vi "terminate.vi"(8 "error in (no error)":errorcluster, 11 "DL090216Display in":refnum<class "DisplayDL090216.lvclass">) -> (0 "error out":errorcluster, 3 "DL090216Display out":refnum<class "DisplayDL090216.lvclass">)   [LabVIEW 2010, in "DisplayDL090216.lvclass"]
uses:
  DisplayDL090216.lvclass
  common/classes/Image/Image/Image.lvclass
  DisplayDL090216.lvclass/DisplayDL090216.ctl
  GenericDisplay/GenericDisplay/GenericDisplay.lvclass
  common/classes/ErrorController/ErrorController/class_data.vi
  common/classes/ErrorController/ErrorController/ErrorController.lvclass
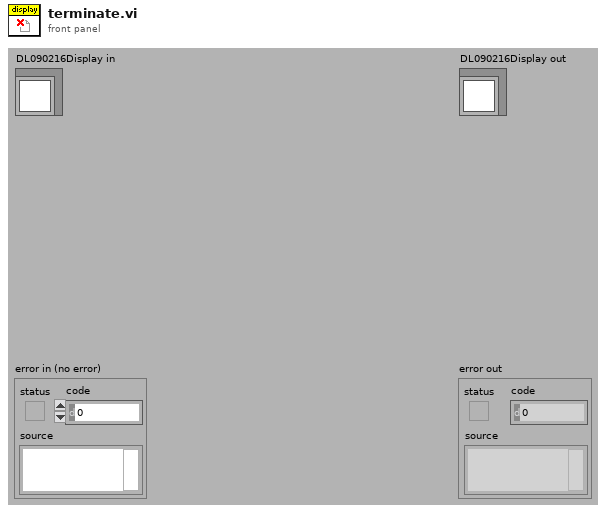
[diagram p1: front panel]
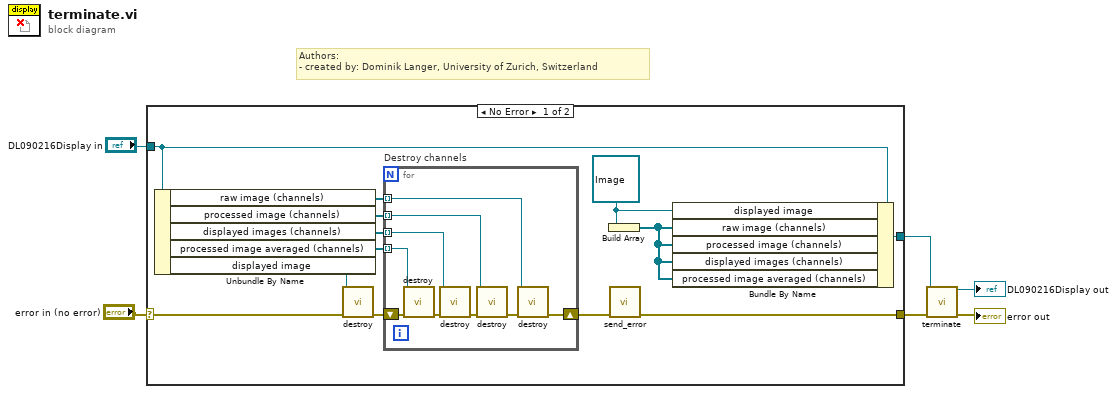
[diagram p0: block diagram]
diagram:
  # "Authors: \n- created by: Dominik Langer, University of Zurich, Switzerland"
  n1 = case shown="No Error" "error in (no error)" {
    selector: "error in (no error)" -> [w10 w30]
    tunnel: [w12 w30] -> w4
    tunnel: [w14 w29] -> w2
    tunnel: "DL090216Display in" -> [w11 w29]
    frame No Error {
      w13 = refnum<class "Image.lvclass"> refnum ("Image.lvclass")
      n2 = Unbundle By Name(w11) -> ("raw image (channels)"=w17:refnum<class "Image.lvclass">[], "processed image (channels)"=w16:refnum<class "Image.lvclass">[], "displayed images (channels)"=w15:refnum<class "Image.lvclass">[], "processed image averaged (channels)"=w8:refnum<class "Image.lvclass">[], "displayed image"=w19:refnum<class "Image.lvclass">)
      n3 = call-dynamic "destroy.vi"("error in (no error)"=w10, "Image in"=w19) -> ("error out"=w18:errorcluster)  [unwired: 9 out]
      n4 = for "Destroy channels" {
        shift-right: [w24] -> w9
        shift-left: w18 -> [w28]
        tunnel: w17 -> [w20] mode=indexing
        tunnel: w16 -> [w21] mode=indexing
        tunnel: w15 -> [w22] mode=indexing
        tunnel: w8 -> [w23] mode=indexing
        n5 = call-dynamic "destroy.vi"("error in (no error)"=w28, "Image in"=w23) -> ("error out"=w27:errorcluster)  [unwired: 9 out]
        n6 = call-dynamic "destroy.vi"("error in (no error)"=w27, "Image in"=w22) -> ("error out"=w26:errorcluster)  [unwired: 9 out]
        n7 = call-dynamic "destroy.vi"("error in (no error)"=w26, "Image in"=w21) -> ("error out"=w25:errorcluster)  [unwired: 9 out]
        n8 = call-dynamic "destroy.vi"("error in (no error)"=w25, "Image in"=w20) -> ("error out"=w24:errorcluster)  [unwired: 9 out]
      }
      n9 = Build Array(w13) -> (w7:refnum<class "Image.lvclass">[])
      n10 = call "send_error.vi"("error in (no error)"=w9) -> ("error out"=w12:errorcluster)  [unwired: 10 in]
      n11 = Bundle By Name(cluster=w11, "displayed image"=w13, "raw image (channels)"=w7, "processed image (channels)"=w7, "displayed images (channels)"=w7, "processed image averaged (channels)"=w7) -> (w14:refnum<class "DisplayDL090216.lvclass">)
    }
    frame Error {
    }
  }
  n12 = call-parent "terminate.vi"("error in (no error)"=w4, "GenericPlugin in"=w2) -> ("error out"=→"error out":errorcluster, "GenericPlugin out"=→"DL090216Display out":refnum<class "DisplayDL090216.lvclass">)  [unwired: 8 out]
